vi "Handle Error.vi"(7 "Stop on Unhandled Error (T)":bool=TRUE, 8 "error in":errorcluster, 11 "RemoteControl.STM":refnum<class "RemoteControl.STM.lvclass">) -> (0 "handling error":errorcluster, 2 "Unhandled error":errorcluster, 3 "RemoteControl.STM out":refnum<class "RemoteControl.STM.lvclass">)   [LabVIEW 2020, in "RemoteControl.STM.lvclass"]
doc: "JKI State Machine Objects (SMO) 1.0.0.11\nJKI - JKI\nCopyright (c) 2016, JKIJKI State Machine Objects (SMO) 1.3.0.56\nJKI - JKI\nCopyright (c) 2017, JKI"
uses:
  RemoteControl.STM.lvclass
  <vilib>/NI/STM/Connection Manager/TCP/TCP Connection Method.ctl
  RemoteControl/RemoteControl.lvclass
  <vilib>/NI/STM/NI STM.lvlib
panel:
  # "For instructions on how to use the JKI State Machine Objects, examples and video tutorials, visit:\nhttp://jki.net/state-machine-objects/\n\nJKI State Machine Objects™\nhttp://jki.net/state-machine-objects/\nCopyright (C) 2005-2015, JKI <info@jki.net>\nALL RIGHTS RESERVED"
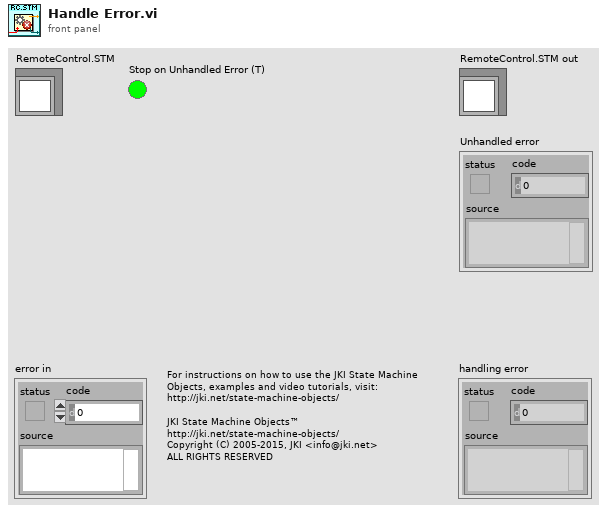
[diagram p1: front panel]
types:
  T1 = typedef "NI STM.lvlib/TCP Connection Method.ctl" = enum16{"Initialize", "Add Connection", "Set Properties", "Get Connection(s)", "Remove Connection", "Remove All Connections", "Get Connection Count"}
  T2 = typedef "NI STM.lvlib/TCP Connection Info.ctl" = cluster{"connection ID":refnum<k5>, "meta data":T3[]}
  T3 = typedef "NI STM.lvlib/MetaDataElement.ctl" = string
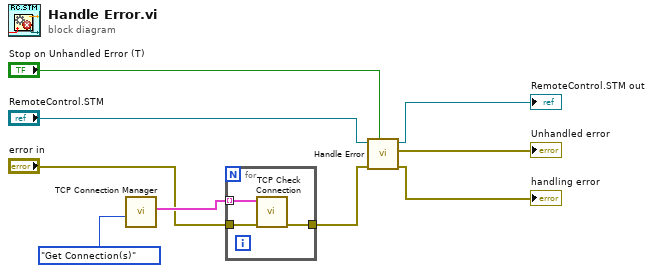
[diagram p0: block diagram]
diagram:
  n1 = call <vilib>:"TCP Connection Manager.vi"("method"=TCP_Connection_Method."Get Connection(s)") -> ("all connections"=w4:T2[])  [unwired: 5 in, 5 out]
  n2 = for {
    tunnel: "error in" -> [w12]
    tunnel: w4 -> [w11] mode=indexing
    tunnel: [w10] -> w1
    n3 = call <vilib>:"TCP Check Connection.vi"("error in"=w12, "connection in"=w11) -> ("error out"=w10:errorcluster)  [unwired: 7 in, 2 out]
  }
  n4 = call-parent "Handle Error.vi"("Stop on Unhandled Error (T)"="Stop on Unhandled Error (T)", "error in"=w1, "LevyLab"="RemoteControl.STM") -> ("handling error"=→"handling error":errorcluster, "Unhandled error"=→"Unhandled error":errorcluster, "LevyLab out"=→"RemoteControl.STM out":refnum<class "RemoteControl.STM.lvclass">)  [unwired: 6 in]
